vi "charts_clear.vi"(8 "error in":errorcluster, 10 "vars general":T1[](array[typedef]) {"stim ramp" min=1}, 11 "control cluster":T3) -> (0 "error out":errorcluster, 2 "vars general":T1[](array[typedef]) {"stim ramp" min=1}, 3 "control cluster":T3)   [LabVIEW 2016]
uses:
  Type Definitions/control_references.ctl
  Type Definitions/vars_settings.ctl
  Type Definitions/stim_type.ctl
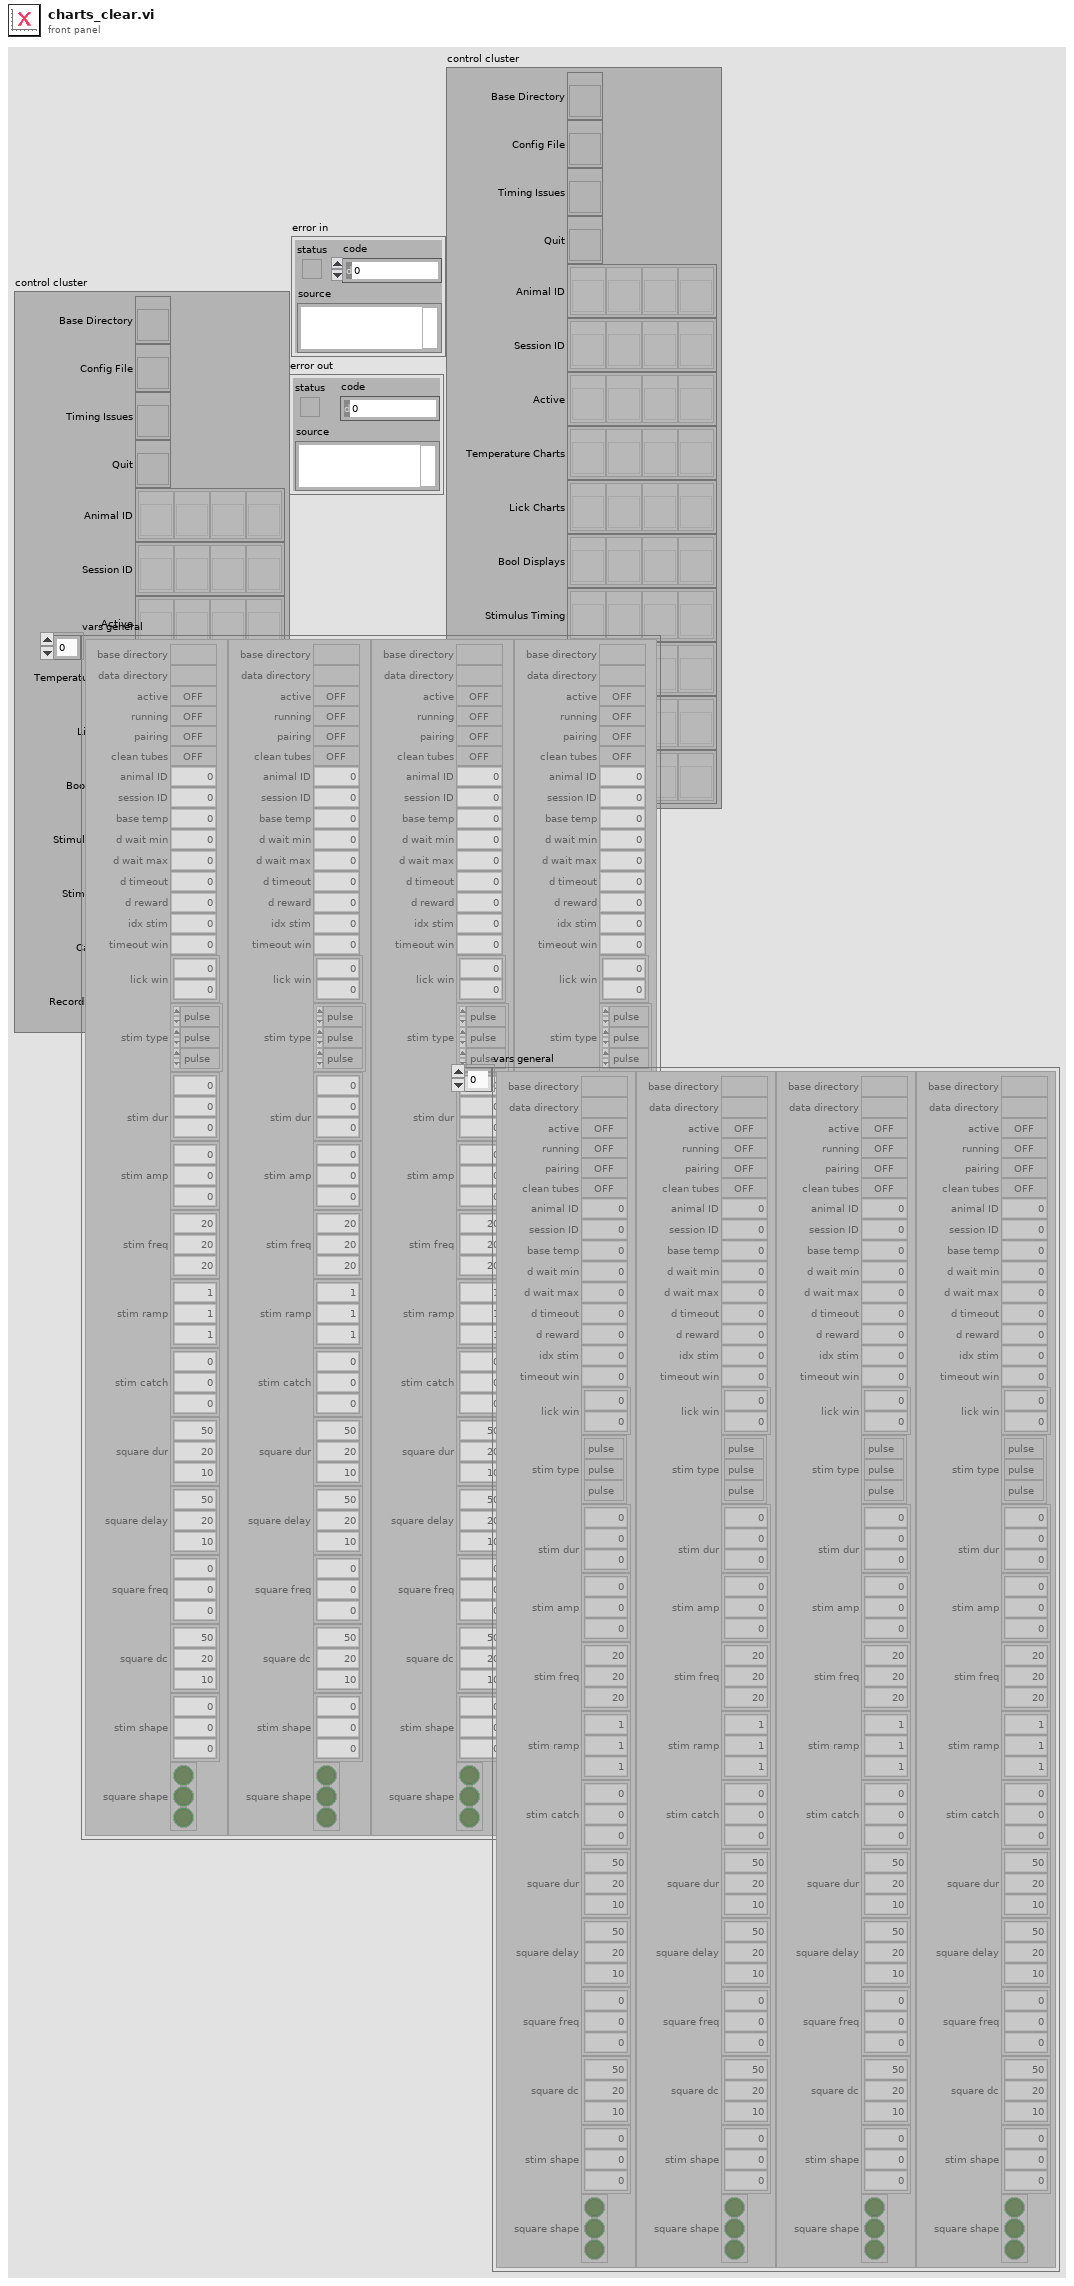
[diagram p1: front panel]
types:
  T1 = typedef "vars_settings.ctl" = cluster{"base directory":path, "data directory":path, "active":bool, "running":bool, "pairing":bool, "clean tubes":bool, "animal ID":u16, "session ID":u16, "base temp":dbl, "d wait min":u16, "d wait max":u16, "d timeout":u16, "d reward":u16, "idx stim":u16, "timeout win":u16, "lick win":i32[], "stim type":T2[], "stim dur":u16[], "stim amp":dbl[], "stim freq":u16[], "stim ramp":u16[], "stim catch":u8[], "square dur":u8[], "square delay":u8[], "square freq":u8[], "square dc":u8[], "stim shape":dbl[][], "square shape":bool[][]}
  T2 = typedef "stim_type.ctl" = enum16{"pulse", "vibration", "square", "sine"}
  T3 = typedef "control_references.ctl" = cluster{"Base Directory":refnum<vi>, "Config File":refnum<vi>, "Timing Issues":refnum<vi>, "Quit":refnum<vi>, "Animal ID":refnum<vi>[], "Session ID":refnum<vi>[], "Active":refnum<vi>[], "Temperature Charts":refnum<vi>[], "Lick Charts":refnum<vi>[], "Bool Displays":refnum<vi>[], "Stimulus Timing":refnum<vi>[], "Stimulus Stats":refnum<vi>[], "Catch Stats":refnum<vi>[], "Recording Status":refnum<vi>[]}
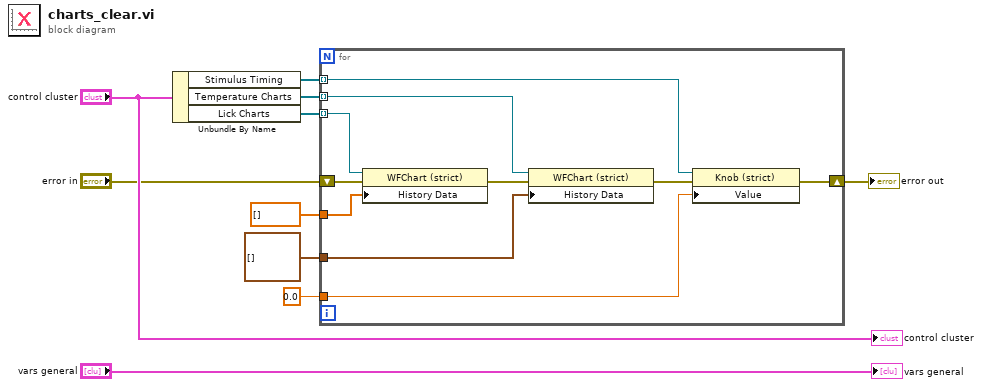
[diagram p0: block diagram]
diagram:
  n1 = Unbundle By Name("control cluster") -> ("Stimulus Timing"=w3:refnum<vi>[], "Temperature Charts"=w5:refnum<vi>[], "Lick Charts"=w4:refnum<vi>[])
  n2 = for {
    shift-right: [w12] -> w10
    shift-left: "error in" -> [w18]
    tunnel: w4 -> [w20] mode=indexing
    tunnel: w5 -> [w15] mode=indexing
    tunnel: dbl[] [] ("History Data") -> [w19]
    tunnel: cluster{"temp in":dbl, "temp in":dbl}[] [] ("History Data") -> [w16]
    tunnel: w3 -> [w13] mode=indexing
    tunnel: 0.0 ("Value") -> [w11]
    n3 = property class="WFChart (strict)"(reference=w20, error in=w18, "History Data"=w19) -> (error out=w17:errorcluster)  [unwired: 1 out]
    n4 = property class="WFChart (strict)"(reference=w15, error in=w17, "History Data"=w16) -> (error out=w14:errorcluster)  [unwired: 1 out]
    n5 = property class="Knob (strict)"(reference=w13, error in=w14, "Value"=w11) -> (error out=w12:errorcluster)  [unwired: 1 out]
  }
  "error out" <- w10
  "control cluster" <- "control cluster"
  "vars general" <- "vars general"
